vi "Add Rock to Chamber.vi"(4 "Rock Position in Chamber in":i32=3, 5 "Rock":u32[][](array[colorbox]), 6 "include Clipped Parts ? (F)":bool, 9 "Chamber in":u32[][](array[colorbox])) -> (0 "Rock Position in Chamber out":i32=3, 3 "Chamber out":u32[][](array[colorbox]))   [LabVIEW 2020, in "AoC 2022.lvlib"]
uses:
  AoC 2022.lvlib
  3ee5d2e5-b28f-4418-a40b-221426a6b43b.vi
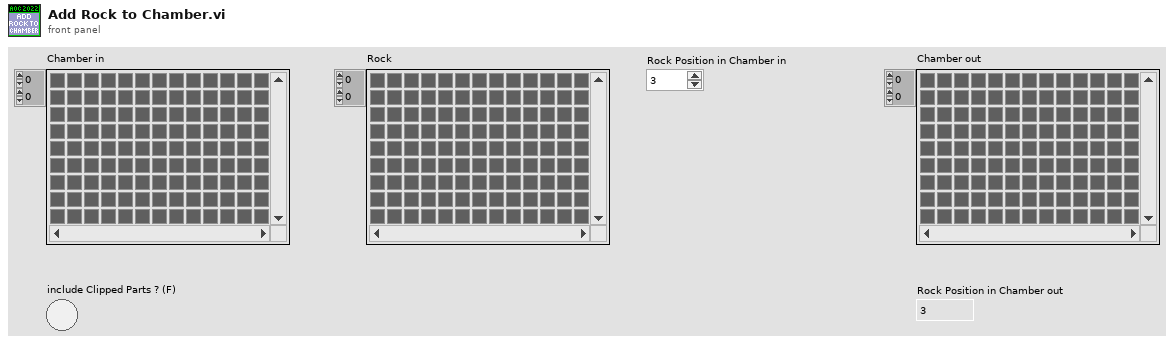
[diagram p1: front panel]
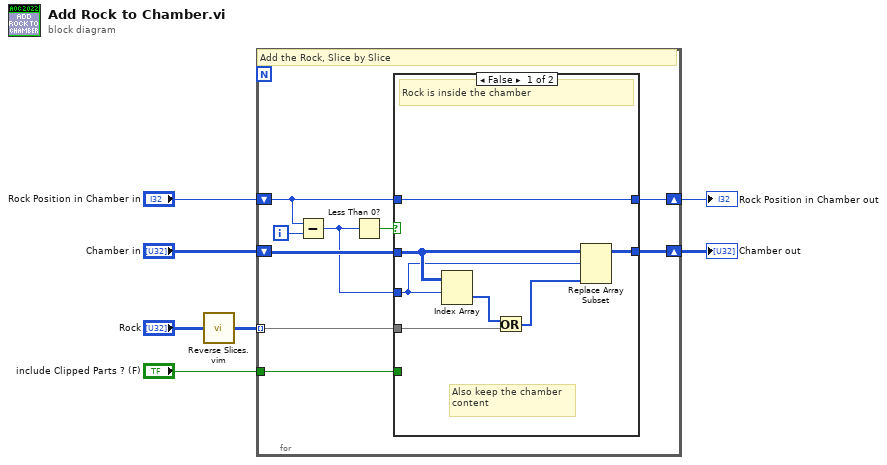
[diagram p0: block diagram]
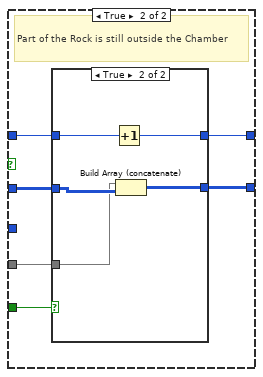
[diagram p2: hidden frame]
diagram:
  n1 = call "Reverse Slices.vim"("Slices"="Rock") -> ("Reversed Slices"=w3:u32[][])
  n2 = for {
    shift-right: [w15] -> w5
    shift-left: "Chamber in" -> [w16]
    tunnel: w3 -> [w14] mode=indexing
    tunnel: "include Clipped Parts ? (F)" -> [w10]
    shift-right: [w8] -> w1
    shift-left: "Rock Position in Chamber in" -> [w9]
    i -> [w13]
    # "Add the Rock, Slice by Slice"
    n3 = Subtract(x=w9, y=w13) -> (x-y=w12:i32)
    n4 = Less Than 0?(x=w12) -> (x < 0?=w11:bool)
    n5 = case shown="False" w11 {
      tunnel: w16 -> [w23 w29]
      tunnel: [w22 w28] -> w15
      tunnel: w14 -> [w21 w27]
      tunnel: w12 -> [w18 _]
      tunnel: w10 -> [_ w26]
      tunnel: w9 -> [w17 w25]
      tunnel: [w17 w24] -> w8
      frame False {
        # "Also keep the chamber content"
        # "Rock is inside the chamber"
        n6 = Index Array(array=w23, index (row)=w18) -> (element=w20:u32[])  [unwired: 1 in]
        n7 = Or(x=w20, y=w21) -> (x .or. y?=w19:u32[])
        n8 = Replace Array Subset(array=w23, new element=w19, index (row)=w18) -> (w22:u32[][])  [unwired: 1 in]
      }
      frame True {
        # "Part of the Rock is still outside the Chamber"
        n9 = case shown="True" w26 {
          tunnel: w29 -> [w31 w36]
          tunnel: [w31 w35] -> w28
          tunnel: w27 -> [_ w34]
          tunnel: w25 -> [w30 w33]
          tunnel: [w30 w32] -> w24
          frame False {
          }
          frame True {
            n10 = Increment(x=w33) -> (x+1=w32:i32)
            n11 = Build Array (concatenate)(w34, w36) -> (w35:u32[][])
          }
        }
      }
    }
  }
  "Chamber out" <- w5
  "Rock Position in Chamber out" <- w1
